vi "partBreal_meantemp.vi"() -> ()   [LabVIEW 2010]
uses:
  <vilib>/Utility/file.llb/Write To Spreadsheet File (DBL).vi
  <vilib>/Analysis/NI_AALBase.lvlib
panel:
  in  "mode (0)":i16
  out "Temp":dbl
  in  "Waittemp":dbl format="%.2f"
  in  "Steptemp":dbl format="%.2f"
  in  "Stopfreq":dbl format="%.2f"
  in  "Startfreq":dbl format="%.2f"
  in  "Stoptemp":dbl format="%.2f"
  in  "Starttemp":dbl format="%.2f"
  out "Numeric 2":dbl format="%.2f"
  in  "Step 2":dbl format="%.2f"
  in  "Stop 2":dbl format="%.2f"
  in  "Start 2":dbl format="%.2f"
  out "data":string
  out "Numeric":dbl format="%.2f"
  out "XY Graph 2":cluster{dbl[], dbl[]}(graph)
  out "XY Graph":cluster{dbl[], dbl[]}(graph)
  in  "Path":path
  out "error out 2":errorcluster
  in  "Wait/s":dbl format="%.2f"
  in  "Stepfreq":dbl format="%.2f"
  in  "error in (no error)":errorcluster
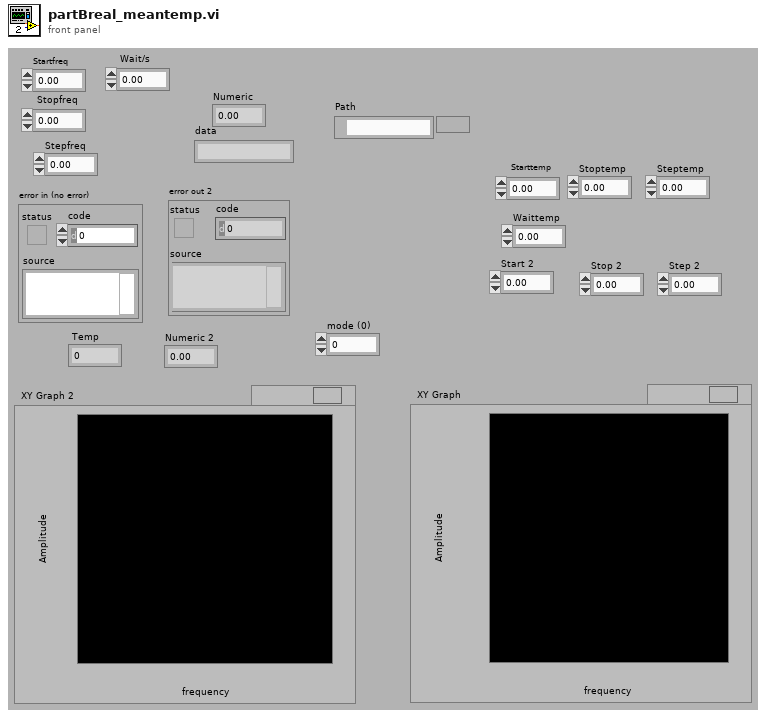
[diagram p1: front panel]
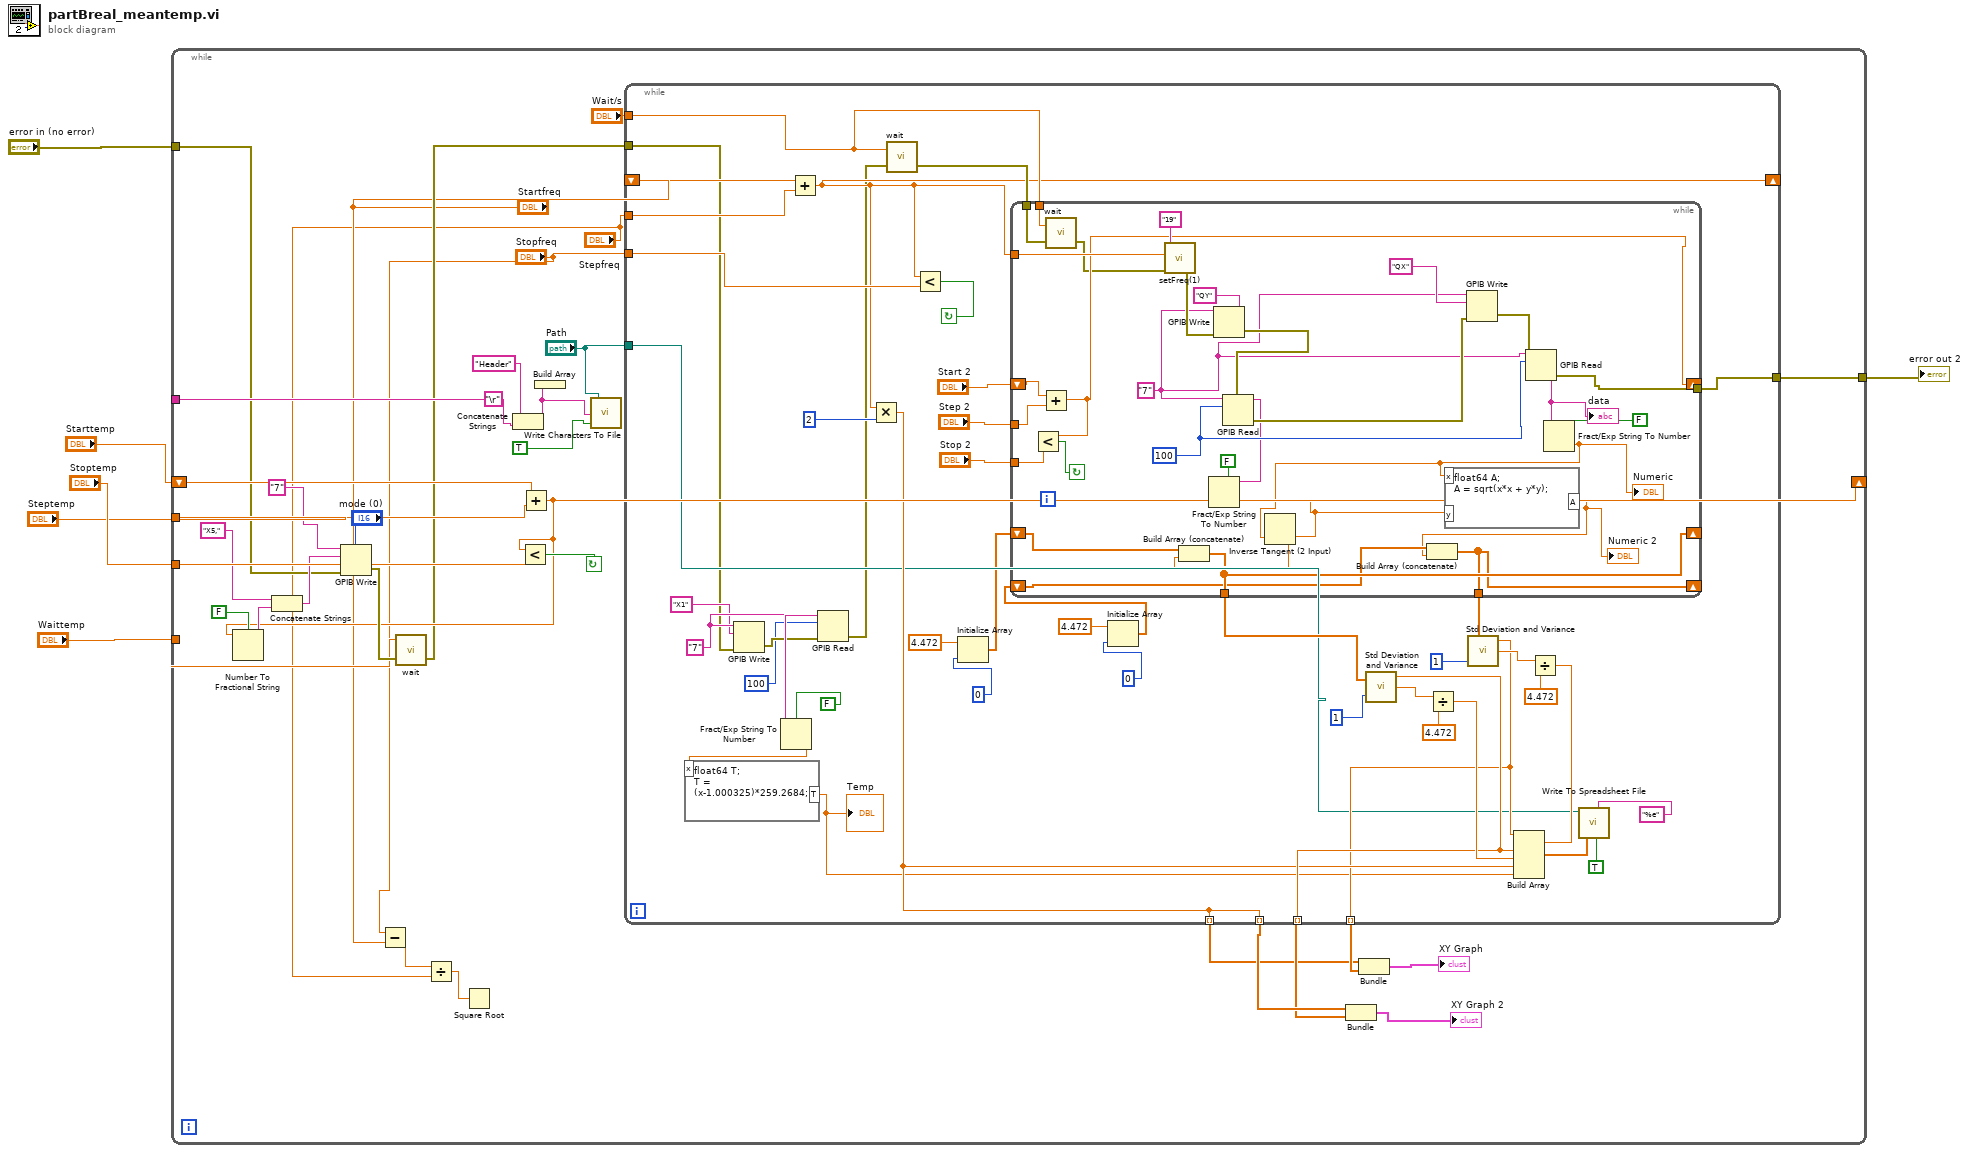
[diagram p0: block diagram]
diagram:
  n1 = while {
    tunnel: "\r" -> [w38]
    tunnel: [w28] -> w6
    shift-right: [w14] -> _
    shift-left: "Starttemp" -> [w27]
    tunnel: "Stoptemp" -> [w25]
    tunnel: "Steptemp" -> [w26]
    tunnel: "Waittemp" -> [w16]
    tunnel: "error in (no error)" -> [w15]
    stop <- w24 continue-if-true
    n2 = Subtract(x="Stopfreq", y="Startfreq") -> (x-y=w11:dbl)
    n3 = Divide(x=w11, y="Stepfreq") -> (x/y=w9:dbl)
    n4 = Square Root(x=w9) -> ()  [unwired: 1 out]
    n5 = Concatenate Strings("Header", w38) -> (w36:string)
    n6 = Add(x=w27, y=w26) -> (x+y=w14:dbl)
    n7 = Number To Fractional String(use system decimal point (T)=FALSE, number=w14) -> (F-format string=w19:string)  [unwired: 2 in]
    n8 = Concatenate Strings("X5,", w19) -> (w17:string)
    n9 = GPIB Write(0:"7", 1:w17, 2:"mode (0)", 3:w15) -> (6:w20:errorcluster)  [unwired: 1 in, 1 out]
    n10 = call "wait.vi"("error in"=w20, "Wartezeit in Sek"=w16) -> ("error out"=w13:errorcluster)  [unwired: 1 in]
    n11 = Less?(x=w14, y=w25) -> (x < y?=w24:bool)
    n12 = Build Array(w36) -> ()  [unwired: 1 out]
    n13 = call <vilib>:"Write Characters To File.vi"("append to file? (new file:F)"=TRUE, "character string"=w36, "file path (dialog if empty)"="Path") -> ()  [unwired: 2 in, 1 out]
    n14 = while {
      tunnel: w13 -> [w43]
      shift-right: [w51] -> _
      shift-left: "Startfreq" -> [w83]
      tunnel: "Stepfreq" -> [w85]
      tunnel: "Stopfreq" -> [w84]
      tunnel: "Wait/s" -> [w61]
      tunnel: "Path" -> [w58]
      tunnel: [w78] -> w28
      tunnel: [w65] -> w32 mode=indexing
      tunnel: [w66] -> w31 mode=indexing
      tunnel: [w65] -> w29 mode=indexing
      tunnel: [w63] -> w30 mode=indexing
      stop <- w82 continue-if-true
      w45 = "7"
      n15 = GPIB Write(0:w45, 1:"X1", 3:w43) -> (6:w48:errorcluster)  [unwired: 2 in, 1 out]
      n16 = Add(x=w83, y=w85) -> (x+y=w51:dbl)
      n17 = GPIB Read(0:w45, 1:100, 3:w48) -> (5:w50:string, 7:w42:errorcluster)  [unwired: 2 in, 1 out]
      n18 = Fract/Exp String To Number(use system decimal point (T)=FALSE, string=w50) -> (number=w49:dbl)  [unwired: 2 in, 1 out]
      n19 = formula code="float64 T;\nT = (x-1.000325)*259.2684;"("x"=w49) -> ("T"=w41:dbl)
      "Temp" <- w41
      n20 = Multiply(x=w51, y=2) -> (x*y=w65:dbl)
      n21 = call "wait.vi"("error in"=w42, "Wartezeit in Sek"=w61) -> ("error out"=w81:errorcluster)  [unwired: 1 in]
      n22 = Less?(x=w51, y=w84) -> (x < y?=w82:bool)
      n23 = Initialize Array(4.472, 0) -> (w55:dbl[])
      n24 = Initialize Array(4.472, 0) -> (w52:dbl[])
      n25 = while {
        tunnel: w81 -> [w94]
        tunnel: w51 -> [w112]
        tunnel: [w107] -> w78
        tunnel: "Step 2" -> [w100]
        tunnel: "Stop 2" -> [w99]
        tunnel: [w88] -> w74
        tunnel: [w90] -> w68
        shift-right: [w96] -> _
        shift-left: "Start 2" -> [w97]
        tunnel: w61 -> [w95]
        shift-right: [w90] -> _
        shift-left: w55 -> [w91]
        shift-right: [w88] -> _
        shift-left: w52 -> [w89]
        stop <- w98 continue-if-true
        w106 = 100
        w108 = "7"
        n26 = Add(x=w97, y=w100) -> (x+y=w96:dbl)
        n27 = Less?(x=w96, y=w99) -> (x < y?=w98:bool)
        n28 = call "wait.vi"("error in"=w94, "Wartezeit in Sek"=w95) -> ("error out"=w93:errorcluster)  [unwired: 1 in]
        n29 = call "setFreq(1).vi"("error in"=w93, "Frequenz in Hz"=w112, "address string"="19") -> ("error out"=w113:errorcluster)  [unwired: 3 in]
        n30 = GPIB Write(0:w108, 1:"QY", 3:w113) -> (6:w114:errorcluster)  [unwired: 2 in, 1 out]
        n31 = GPIB Read(0:w108, 1:w106, 3:w114) -> (5:w104:string, 7:w110:errorcluster)  [unwired: 2 in, 1 out]
        n32 = Fract/Exp String To Number(use system decimal point (T)=FALSE, string=w104) -> (number=w105:dbl)  [unwired: 2 in, 1 out]
        n33 = GPIB Write(0:w108, 1:"QX", 3:w110) -> (6:w109:errorcluster)  [unwired: 2 in, 1 out]
        n34 = GPIB Read(0:w108, 1:w106, 3:w109) -> (5:w102:string, 7:w107:errorcluster)  [unwired: 2 in, 1 out]
        "data" <- w102
        n35 = Fract/Exp String To Number(use system decimal point (T)=FALSE, string=w102) -> (number=w103:dbl)  [unwired: 2 in, 1 out]
        "Numeric" <- w103
        n36 = Inverse Tangent (2 Input)(1:w103, 2:w105) -> (0:w92:dbl)
        n37 = Build Array (concatenate)(w91, w92) -> (w90:dbl[])
        n38 = formula code="float64 A;\nA = sqrt(x*x + y*y);"("x"=w103, "y"=w105) -> ("A"=w87:dbl)
        "Numeric 2" <- w87
        n39 = Build Array (concatenate)(w89, w87) -> (w88:dbl[])
      }
      n40 = call <vilib>:"Std Deviation and Variance.vi"("X"=w68, "Weighting (Sample)"=1) -> ("mean"=w66:dbl, "standard deviation"=w70:dbl)  [unwired: 1 out]
      n41 = Divide(x=w70, y=4.472) -> (x/y=w67:dbl)
      n42 = call <vilib>:"Std Deviation and Variance.vi"("X"=w74, "Weighting (Sample)"=1) -> ("mean"=w63:dbl, "standard deviation"=w73:dbl)  [unwired: 1 out]
      n43 = Divide(x=w73, y=4.472) -> (x/y=w71:dbl)
      n44 = Build Array(w63, w71, w66, w67, w65, w41) -> (w64:dbl[])
      n45 = call-poly <vilib>:"Write To Spreadsheet File.vi"("format (%.3f)"="%e", "append to file? (new file:F)"=TRUE, "1D data"=w64, "file path (dialog if empty)"=w58) -> ()  [unwired: 4 in, 1 out]
    }
    n46 = Bundle(w32, w31) -> (→"XY Graph 2":cluster{dbl[], dbl[]})  [unwired: 1 in]
    n47 = Bundle(w29, w30) -> (→"XY Graph":cluster{dbl[], dbl[]})  [unwired: 1 in]
  }
  "error out 2" <- w6
